vi "Get LabVIEW File Version.vi"(8 "Error In":errorcluster, 11 "File Path Control":path) -> (0 "Error Out":errorcluster, 2 "Version":string, 3 "Duplicate Path":path)   [LabVIEW 2020, in "LMH-Toolbox.lvlib"]
uses:
  LMH-Toolbox.lvlib
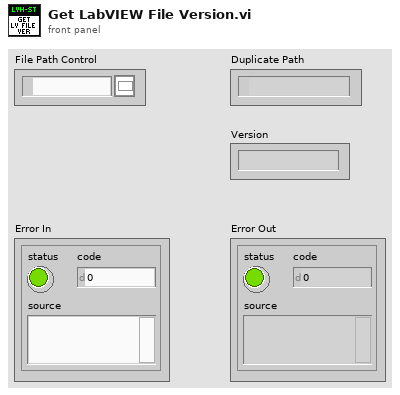
[diagram p1: front panel]
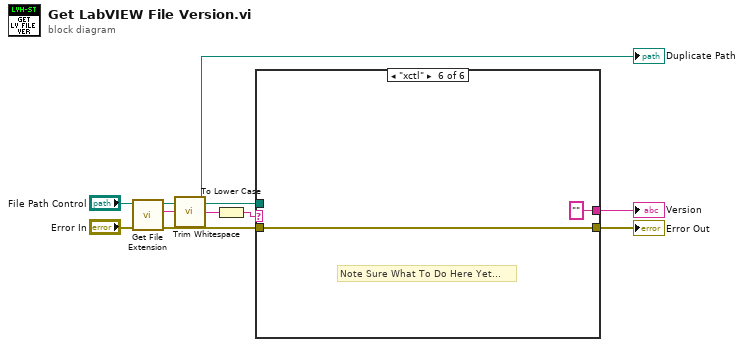
[diagram p0: block diagram]
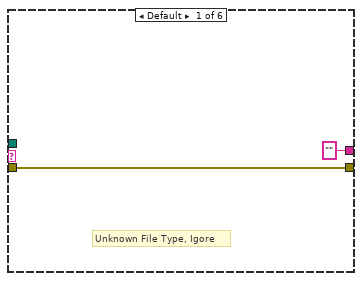
[diagram p2: hidden frame]
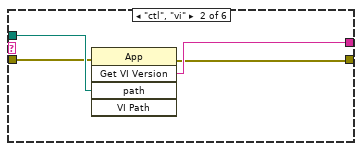
[diagram p3: hidden frame]
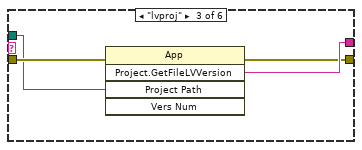
[diagram p4: hidden frame]
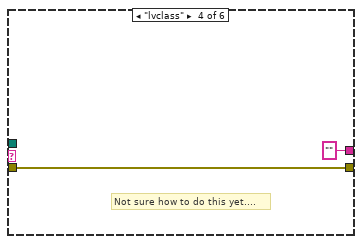
[diagram p5: hidden frame]
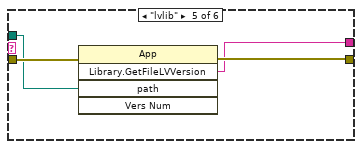
[diagram p6: hidden frame]
diagram:
  n1 = call "Get File Extension.vi"("Error In"="Error In", "File Path Control"="File Path Control") -> ("Error Out"=w7:errorcluster, "Extension"=w5:string, "Duplicate Path"=w1:path)  [unwired: 7 in]
  "Duplicate Path" <- w1
  n2 = call <vilib>:"Trim Whitespace.vi"("string"=w5) -> ("trimmed string"=w6:string)  [unwired: 1 in]
  n3 = To Lower Case(string=w6) -> (all lower case string=w4:string)
  n4 = case shown="\"xctl\"" w4 {
    tunnel: w1 -> [_ w15 w16 _ w23 _]
    tunnel: w7 -> [w10 w13 w19 w21 w25 w27]
    tunnel: ["" ("Project.GetFileLVVersion") w14 w18 "" ("Project.GetFileLVVersion") w22 "" ("Library.GetFileLVVersion")] -> w3
    tunnel: [w10 w12 w17 w21 w24 w27] -> w2
    frame Default {
      # "Unknown File Type, Igore"
    }
    frame "ctl", "vi" {
      n5 = invoke class="App" method="Get VI Version"(error in=w13, "path"=w15) -> (error out=w12:errorcluster, "GetVIVers"=w14:string)  [unwired: 3 in, 3 out]
    }
    frame "lvproj" {
      n6 = invoke class="App" method="Project.GetFileLVVersion"(error in=w19, "Project Path"=w16) -> (error out=w17:errorcluster, "Project.GetFileLVVersion"=w18:string)  [unwired: 3 in, 3 out]
    }
    frame "lvclass" {
      # "Not sure how to do this yet...."
    }
    frame "lvlib" {
      n7 = invoke class="App" method="Library.GetFileLVVersion"(error in=w25, "path"=w23) -> (error out=w24:errorcluster, "Library.GetFileLVVersion"=w22:string)  [unwired: 3 in, 3 out]
    }
    frame "xctl" {
      # "Note Sure What To Do Here Yet..."
    }
  }
  "Error Out" <- w2
  "Version" <- w3
